vi "String_Type_Checker.vi"(11 "String":string) -> (1 "Number":string, 3 "Type":string)   [LabVIEW 2025, in "Table_Filtering.lvlib"]
uses:
  Table_Filtering.lvlib
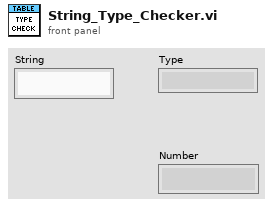
[diagram p1: front panel]
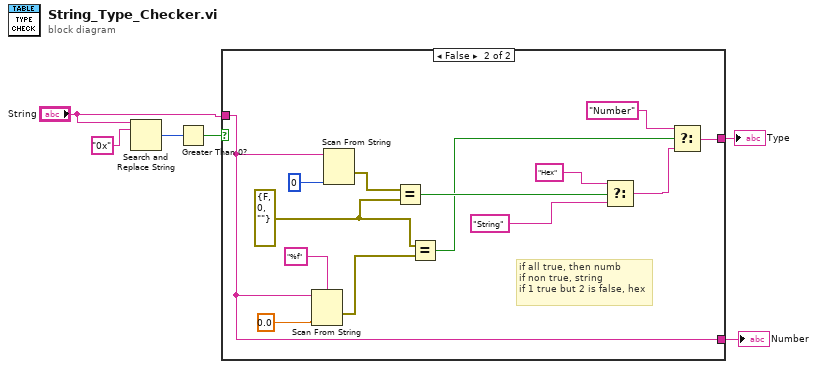
[diagram p0: block diagram]
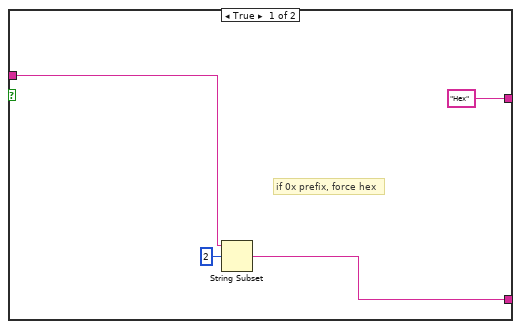
[diagram p2: hidden frame]
diagram:
  n1 = Search and Replace String(input string="String", search string="0x" ("regular expression")) -> (number of replacements=w4:i32)  [unwired: 6 in, 3 out]
  n2 = Greater Than 0?(x=w4) -> (x > 0?=w3:bool)
  n3 = case shown="False" w3 {
    tunnel: ["Hex" ("t") w19] -> w6
    tunnel: "String" -> [w9 w20]
    tunnel: [w7 w20] -> w2
    frame True {
      # "if 0x prefix, force hex"
      n4 = String Subset(string=w9, offset (0)=2) -> (substring=w7:string)  [unwired: 1 in]
    }
    frame False {
      w13 = errorcluster {"status"=FALSE, "code"=0, "source"=""} ("error constant")
      # "if all true, then numb\nif non true, string\nif 1 true but 2 is false, hex"
      n5 = Scan From String(format string="%f", input string=w20, default 1=0.0 ("default value 1")) -> (error out=w14:errorcluster)  [unwired: 3 in, 2 out]
      n6 = Scan From String(input string=w20, default 1=u32 0 ("default value 1")) -> (error out=w15:errorcluster)  [unwired: 4 in, 2 out]
      n7 = Equal?(x=w15, y=w13) -> (x = y?=w12:bool)
      n8 = Equal?(x=w13, y=w14) -> (x = y?=w11:bool)
      n9 = Select(t="Hex", s=w12, f="String") -> (s? t:f=w23:string)
      n10 = Select(t="Number", s=w11, f=w23) -> (s? t:f=w19:string)
    }
  }
  "Type" <- w6
  "Number" <- w2
